vi "done.vi"(7 "waitgroup":T1, 8 "error in (no error)":errorcluster, 10 "child_id":T2, 11 "queue":refnum<queue>) -> (0 "error out":errorcluster)   [LabVIEW 2015, in "lv-waitgroup.lvlib"]
uses:
  lv-waitgroup.lvlib
  _controls/api_child_queue.ctl
  _controls/api_waitgroup.ctl
  private/_controls/waitgroup.ctl
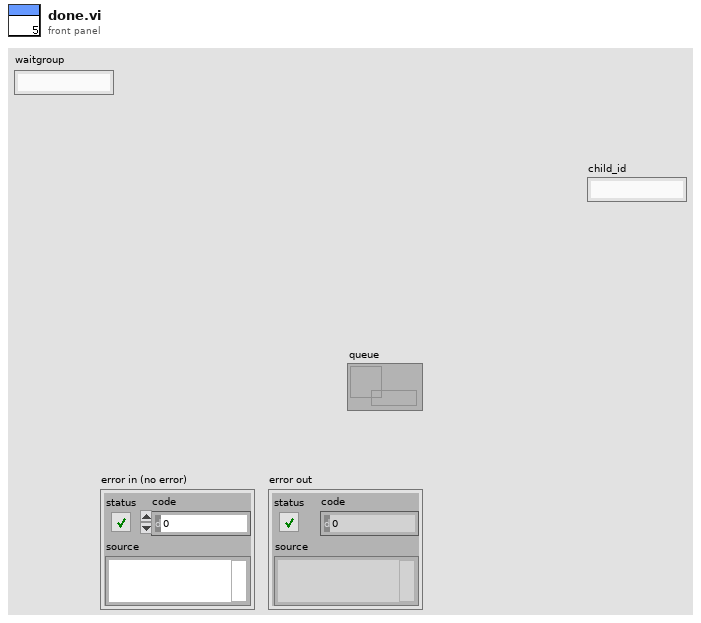
[diagram p1: front panel]
types:
  T1 = typedef "lv-waitgroup.lvlib/api_waitgroup.ctl" = string
  T2 = typedef "lv-waitgroup.lvlib/api_child_queue.ctl" = string
  T3 = typedef "lv-waitgroup.lvlib/waitgroup.ctl" = cluster{"waitgroup":refnum<queue>, "queues":variant}
  T4 = typedef "lv-waitgroup.lvlib/references.ctl" = cluster{"waitgroups":refnum<data-value>}
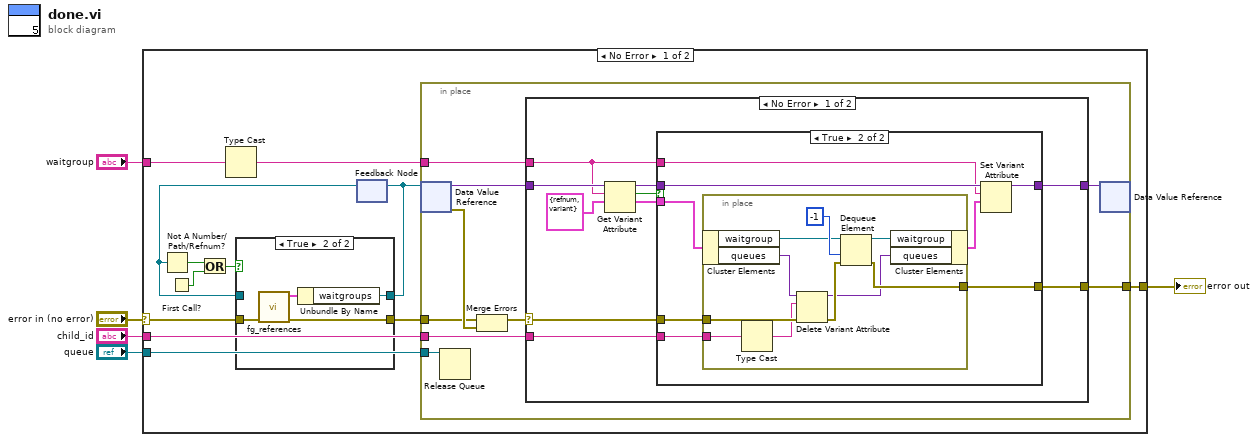
[diagram p0: block diagram]
diagram:
  n1 = case shown="No Error" "error in (no error)" {
    selector: "error in (no error)" -> [w7 w65]
    tunnel: "waitgroup" -> [w10 _]
    tunnel: "queue" -> [w17 _]
    tunnel: "child_id" -> [w16 _]
    tunnel: [w15 w65] -> w1
    frame No Error {
      n2 = First Call?() -> (First Call?: T/F=w12:bool)
      n3 = Type Cast(x=w10) -> (*(type *) &x=w9:string)  [unwired: 1 in]
      n4 = feedback #1() -> (w11:refnum<data-value>)  [unwired: 1 in]
      n5 = Not A Number/Path/Refnum?(number/path/refnum=w11) -> (NaN/Path/Refnum?=w14:bool)
      n6 = Or(x=w14, y=w12) -> (x .or. y?=w13:bool)
      n7 = case shown="True" w13 {
        tunnel: w7 -> [w18 w23]
        tunnel: [w18 w21] -> w6
        tunnel: [w19 w20] -> w8
        tunnel: w11 -> [w19 _]
        frame False {
        }
        frame True {
          n8 = call "fg_references.vi"("error in (no error)"=w23) -> ("error out"=w21:errorcluster, "references out"=w22:T4)  [unwired: 9 in]
          n9 = Unbundle By Name(w22) -> ("waitgroups"=w20:refnum<data-value>)
        }
      }
      n10 = feedback-in #1(w8) -> ()
      n11 = in-place {
        in-place-border: w9 -> [w26]
        in-place-border: w6 -> [w30]
        in-place-border: w17 -> [w29]
        in-place-border: w16 -> [w28]
        in-place-border: [w24] -> w15
        n12 = in-place-dvr #2(w8) -> (w32:variant, w31:errorcluster)
        n13 = Release Queue(queue=w29) -> ()  [unwired: 2 in, 3 out]
        n14 = Merge Errors(w30, w31) -> (w25:errorcluster)
        n15 = case shown="No Error" w25 {
          selector: w25 -> [w35 w64]
          tunnel: w32 -> [w42 w63]
          tunnel: w28 -> [w40 _]
          tunnel: [w37 w63] -> w27
          tunnel: w26 -> [w36 _]
          tunnel: [w34 w64] -> w24
          frame No Error {
            n16 = Get Variant Attribute(Variant=w42, name=w36, default value (empty Variant)=T3 {"waitgroup"=refnum, "queues"=variant} ("shared_data")) -> (duplicate Variant=w38:variant, found=w33:bool, value=w39:T3)  [unwired: 1 in, 1 out]
            n17 = case shown="True" w33 {
              tunnel: w40 -> [_ w52]
              tunnel: w39 -> [_ w51]
              tunnel: w38 -> [w44 w50]
              tunnel: [w44 w49] -> w37
              tunnel: w36 -> [_ w48]
              tunnel: w35 -> [w43 w46]
              tunnel: [w43 w45] -> w34
              frame False {
              }
              frame True {
                n18 = in-place {
                  in-place-border: w52 -> [w54]
                  in-place-border: w46 -> [w62]
                  in-place-border: [w59] -> w45
                  n19 = in-place-cluster #3(w51) -> ("waitgroup"=w58:refnum<queue>, "queues"=w55:variant)
                  n20 = Type Cast(x=w54) -> (*(type *) &x=w53:string)  [unwired: 1 in]
                  n21 = Delete Variant Attribute(4:w62, 6:w53, 7:w55) -> (0:w61:errorcluster, 3:w56:variant)  [unwired: 1 out]
                  n22 = Dequeue Element(queue=w58, timeout in ms (-1)=-1, error in (no error)=w61) -> (queue out=w57:refnum<queue>, error out=w59:errorcluster)  [unwired: 2 out]
                  n23 = in-place-cluster #3("waitgroup"=w57, "queues"=w56) -> (w47:T3)
                }
                n24 = Set Variant Attribute(Variant=w50, name=w48, value=w47) -> (Variant out=w49:variant)  [unwired: 1 in, 2 out]
              }
            }
          }
          frame Error {
          }
        }
        n25 = in-place-dvr #2(w27) -> ()  [unwired: 2 out]
      }
    }
    frame Error {
    }
  }
  "error out" <- w1
